vi "generic_test.vi"() -> ()   [LabVIEW 2011]
uses:
  C:/OmniDriverSPAM/OOI_HOME/NETOmniDriver-NET20.dll
  OmniDriverSPAM/OOI_HOME/NETOmniDriver-NET20.dll
panel:
  out "TEC Error Log":errorcluster
  in  "TEC Setpoint [°C]":dbl=-15.0
  out "getSpectrum Times Array":u32[](array[numeric])
  in  "ExtraDelay After Loop":bool
  in  "LoopExit":bool
  out "getSpectrumTime [ms]":u32
  in  "Trigger Mode":i32
  out "Spectrometer Type":string
  out "XY Graph":cluster{"Y":dbl[], "Y":dbl[]}[](graph) caption="XY-Graph"
  out "Spectrum":dbl[](array[numeric])
  out "Wavelengths [nm]":dbl[](array[numeric])
  in  "Scans to Average":i32=1
  in  "Int. Time [ms]":i32=1000
  out "MinIntTime [ms]":i32
  out "NETWrapper\nStatus":errorcluster caption="NETWrapper Status"
  out "MaxIntTime [ms]":i32
  in  "spectrometerIndex":i32
  out "Serial\nNumber":string
  out "Number attached\nSpectrometers":i32
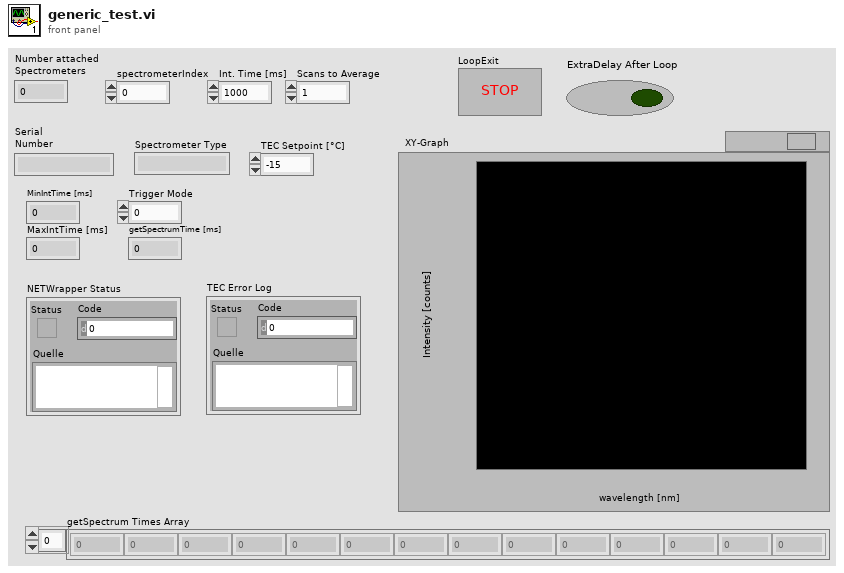
[diagram p1: front panel]
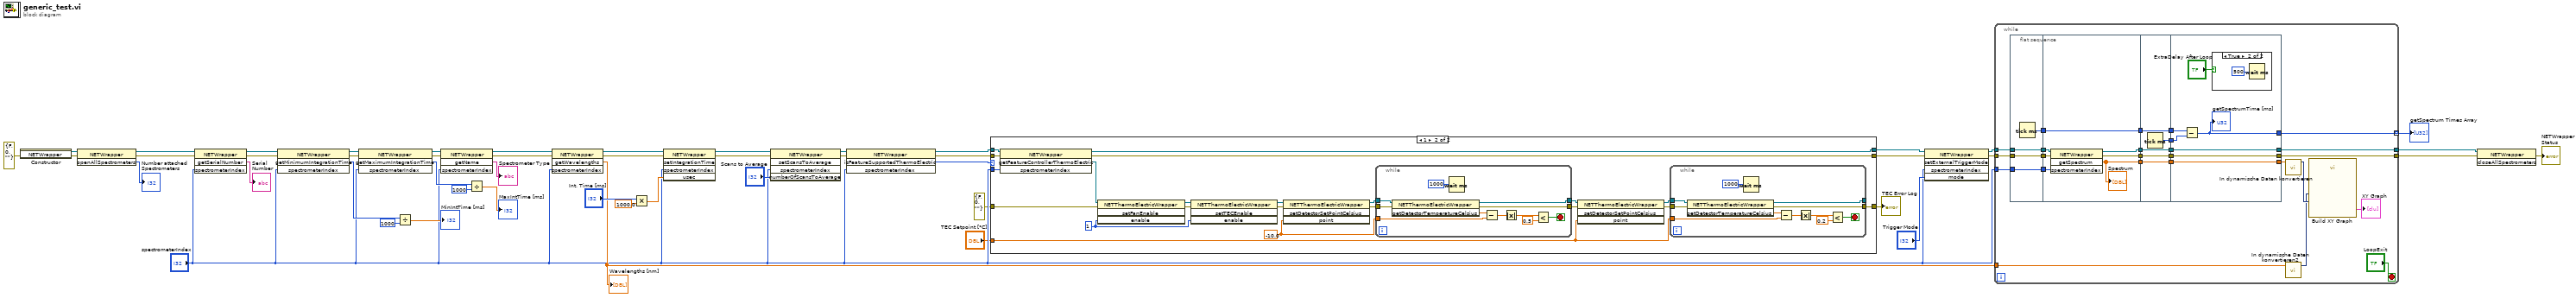
[diagram p0: block diagram]
diagram:
  n1 = constructor class="NETWrapper"(error in=errorcluster {"status"=FALSE, "code"=0, "source"=""} ("Fehler (Eingang, kein Fehler)")) -> (reference out=w14:refnum<k24>, error out=w13:errorcluster)  [unwired: 2 in, 1 out]
  n2 = invoke class="NETWrapper" method="openAllSpectrometers"(reference=w14, error in=w13) -> (reference out=w48:refnum<k24>, error out=w47:errorcluster, "openAllSpectrometers"=→"Number attached\nSpectrometers":i32)  [unwired: 1 in]
  n3 = invoke class="NETWrapper" method="getSerialNumber"(reference=w48, error in=w47, "spectrometerIndex"="spectrometerIndex") -> (reference out=w45:refnum<k24>, error out=w44:errorcluster, "getSerialNumber"=→"Serial\nNumber":string)  [unwired: 1 in, 1 out]
  n4 = invoke class="NETWrapper" method="getMinimumIntegrationTime"(reference=w45, error in=w44, "spectrometerIndex"="spectrometerIndex") -> (reference out=w43:refnum<k24>, error out=w42:errorcluster, "getMinimumIntegrationTime"=w38:i32)  [unwired: 1 in, 1 out]
  n5 = invoke class="NETWrapper" method="getMaximumIntegrationTime"(reference=w43, error in=w42, "spectrometerIndex"="spectrometerIndex") -> (reference out=w22:refnum<k24>, error out=w24:errorcluster, "getMaximumIntegrationTime"=w23:i32)  [unwired: 1 in, 1 out]
  n6 = Divide(x=w38, y=1000) -> (x/y=→"MinIntTime [ms]":dbl)
  n7 = invoke class="NETWrapper" method="getName"(reference=w22, error in=w24, "spectrometerIndex"="spectrometerIndex") -> (reference out=w20:refnum<k24>, error out=w19:errorcluster, "getName"=→"Spectrometer Type":string)  [unwired: 1 in, 1 out]
  n8 = Divide(x=w23, y=1000) -> (x/y=→"MaxIntTime [ms]":dbl)
  n9 = invoke class="NETWrapper" method="getWavelengths"(reference=w20, error in=w19, "spectrometerIndex"="spectrometerIndex") -> (reference out=w29:refnum<k24>, error out=w28:errorcluster, "getWavelengths"=w25:dbl[])  [unwired: 1 in, 1 out]
  "Wavelengths [nm]" <- w25
  n10 = Multiply(x="Int. Time [ms]", y=1000.0) -> (x*y=w35:dbl)
  n11 = invoke class="NETWrapper" method="setIntegrationTime"(reference=w29, error in=w28, "spectrometerIndex"="spectrometerIndex", "usec"=w35) -> (reference out=w31:refnum<k24>, error out=w32:errorcluster)  [unwired: 1 in, 3 out]
  n12 = invoke class="NETWrapper" method="setScansToAverage"(reference=w31, error in=w32, "spectrometerIndex"="spectrometerIndex", "numberOfScansToAverage"="Scans to Average") -> (reference out=w5:refnum<k24>, error out=w3:errorcluster)  [unwired: 1 in, 3 out]
  n13 = invoke class="NETWrapper" method="isFeatureSupportedThermoElectric"(reference=w5, error in=w3, "spectrometerIndex"="spectrometerIndex") -> (reference out=w9:refnum<k24>, error out=w8:errorcluster, "isFeatureSupportedThermoElectric"=w11:i16)  [unwired: 1 in, 1 out]
  n14 = case shown="1" w11 {
    tunnel: "spectrometerIndex" -> [_ w73]
    tunnel: w9 -> [w52 w72]
    tunnel: w8 -> [w51 w71]
    tunnel: errorcluster {"status"=FALSE, "code"=0, "source"=""} ("Fehler (Eingang, kein Fehler)") -> [w50 w69]
    tunnel: "TEC Setpoint [°C]" -> [_ w58]
    tunnel: [w51 w55] -> w2
    tunnel: [w52 w54] -> w4
    tunnel: [w50 w53] -> w1
    frame 0, Default {
    }
    frame 1 {
      w61 = -10.0 ("point")
      w66 = i16 1 ("enable")
      n15 = invoke class="NETWrapper" method="getFeatureControllerThermoElectric"(reference=w72, error in=w71, "spectrometerIndex"=w73) -> (reference out=w54:refnum<k24>, error out=w55:errorcluster, "getFeatureControllerThermoElectric"=w70:refnum<k24>)  [unwired: 1 in, 1 out]
      n16 = invoke class="NETThermoElectricWrapper" method="setFanEnable"(reference=w70, error in=w69, "enable"=w66) -> (reference out=w67:refnum<k24>, error out=w68:errorcluster)  [unwired: 1 in, 2 out]
      n17 = invoke class="NETThermoElectricWrapper" method="setTECEnable"(reference=w67, error in=w68, "enable"=w66) -> (reference out=w65:refnum<k24>, error out=w64:errorcluster)  [unwired: 1 in, 2 out]
      n18 = invoke class="NETThermoElectricWrapper" method="setDetectorSetPointCelsius"(reference=w65, error in=w64, "point"=w61) -> (reference out=w62:refnum<k24>, error out=w63:errorcluster)  [unwired: 1 in, 2 out]
      n19 = while {
        tunnel: w63 -> [w95]
        tunnel: w62 -> [w94]
        tunnel: w61 -> [w91]
        tunnel: [w86] -> w60
        tunnel: [w85] -> w59
        stop <- w87 stop-if-true
        n20 = invoke class="NETThermoElectricWrapper" method="getDetectorTemperatureCelsius"(reference=w94, error in=w95) -> (reference out=w85:refnum<k24>, error out=w86:errorcluster, "getDetectorTemperatureCelsius"=w92:dbl)  [unwired: 1 in]
        n21 = Wait (ms)(milliseconds to wait=u32 1000 ("Zu wartende ms")) -> ()  [unwired: 1 out]
        n22 = Subtract(x=w92, y=w91) -> (x-y=w89:dbl)
        n23 = Absolute Value(x=w89) -> (abs(x)=w90:dbl)
        n24 = Less?(x=w90, y=0.5) -> (x < y?=w87:bool)
      }
      n25 = invoke class="NETThermoElectricWrapper" method="setDetectorSetPointCelsius"(reference=w59, error in=w60, "point"=w58) -> (reference out=w57:refnum<k24>, error out=w56:errorcluster)  [unwired: 1 in, 2 out]
      n26 = while {
        tunnel: w56 -> [w84]
        tunnel: w57 -> [w83]
        tunnel: w58 -> [w80]
        tunnel: [w75] -> w53
        tunnel: [w74] -> _
        stop <- w76 stop-if-true
        n27 = invoke class="NETThermoElectricWrapper" method="getDetectorTemperatureCelsius"(reference=w83, error in=w84) -> (reference out=w74:refnum<k24>, error out=w75:errorcluster, "getDetectorTemperatureCelsius"=w81:dbl)  [unwired: 1 in]
        n28 = Wait (ms)(milliseconds to wait=u32 1000 ("Zu wartende ms")) -> ()  [unwired: 1 out]
        n29 = Subtract(x=w81, y=w80) -> (x-y=w78:dbl)
        n30 = Absolute Value(x=w78) -> (abs(x)=w79:dbl)
        n31 = Less?(x=w79, y=0.2) -> (x < y?=w76:bool)
      }
    }
  }
  "TEC Error Log" <- w1
  n32 = invoke class="NETWrapper" method="setExternalTriggerMode"(reference=w4, error in=w2, "spectrometerIndex"="spectrometerIndex", "mode"="Trigger Mode") -> (reference out=w18:refnum<k24>, error out=w17:errorcluster)  [unwired: 1 in, 3 out]
  n33 = while {
    tunnel: w18 -> [w120]
    tunnel: [w119] -> w27
    tunnel: [w118] -> w26
    tunnel: w25 -> [w114]
    tunnel: "spectrometerIndex" -> [w112]
    tunnel: w17 -> [w111]
    tunnel: [w96] -> w15 mode=indexing
    stop <- "LoopExit" stop-if-true
    n34 = flat-sequence {
      tunnel: w111 -> [w122]
      tunnel: w112 -> [w123]
      tunnel: w120 -> [w124]
      tunnel: [w124] -> w110
      tunnel: [w123] -> w109
      tunnel: [w122] -> w108
      tunnel: [w121] -> w100
      tunnel: w110 -> [w131]
      tunnel: w109 -> [w128]
      tunnel: w108 -> [w127]
      tunnel: [w130] -> w107
      tunnel: [w129] -> w106
      tunnel: [w126] -> w105
      tunnel: w100 -> [w125]
      tunnel: [w125] -> w99
      tunnel: w107 -> [w136]
      tunnel: w106 -> [w135]
      tunnel: w105 -> [w134]
      tunnel: [w136] -> w104
      tunnel: [w135] -> w103
      tunnel: [w134] -> w102
      tunnel: [w133] -> w101
      tunnel: w99 -> [w132]
      tunnel: [w132] -> w98
      tunnel: [w141] -> w116
      tunnel: [w142] -> w118
      tunnel: [w143] -> w119
      tunnel: w104 -> [w143]
      tunnel: w103 -> [w142]
      tunnel: w102 -> [w141]
      tunnel: w101 -> [w140]
      tunnel: w98 -> [w139]
      tunnel: [w137] -> w96
      frame #0 {
        n35 = Tick Count (ms)() -> (millisecond timer value=w121:u32)
      }
      frame #1 {
        n36 = invoke class="NETWrapper" method="getSpectrum"(reference=w131, error in=w127, "spectrometerIndex"=w128) -> (reference out=w130:refnum<k24>, error out=w129:errorcluster, "getSpectrum"=w126:dbl[])  [unwired: 1 in, 1 out]
        "Spectrum" <- w126
      }
      frame #2 {
        n37 = Tick Count (ms)() -> (millisecond timer value=w133:u32)
      }
      frame #3 {
        n38 = Subtract(x=w139, y=w140) -> (x-y=w137:u32)
        "getSpectrumTime [ms]" <- w137
        n39 = case shown="True" "ExtraDelay After Loop" {
          frame False {
          }
          frame True {
            n40 = Wait (ms)(milliseconds to wait=u32 500 ("Zu wartende ms")) -> ()  [unwired: 1 out]
          }
        }
      }
    }
    n41 = call "In dynamische Daten konvertieren"("Array"=w116) -> ("Dynamic Data Type"=w115:dynamicdata)  [unwired: 3 in]
    n42 = call "In dynamische Daten konvertieren2"("Array"=w114) -> ("Dynamic Data Type"=w113:dynamicdata)  [unwired: 3 in]
    n43 = call "Build XY Graph"("Y Input"=w115, "X Input"=w113) -> ("XY Graph"=→"XY Graph":cluster{"Y":dbl[], "Y":dbl[]}[])  [unwired: 3 in, 6 out]
  }
  "getSpectrum Times Array" <- w15
  n44 = invoke class="NETWrapper" method="closeAllSpectrometers"(reference=w27, error in=w26) -> (error out=→"NETWrapper\nStatus":errorcluster)  [unwired: 1 in, 2 out]
